vi "Get Broadcast Event.vi"(8 "error in (no error)":errorcluster, 11 "Debug View In":refnum<class "Debug View.lvclass">) -> (0 "error out":errorcluster, 2 "Broadcast Event":refnum<user-event>[](array[refnum]), 3 "Debug View Out":refnum<class "Debug View.lvclass">)   [LabVIEW 2020, in "Debug View.lvclass"]
doc: "Get the broadcast event used to send broadcasts to registered observers."
uses:
  Debug View.lvclass
  Protected/Broadcasting/Broadcast Message Cluster.ctl
  Debug View.lvclass/Debug View.ctl
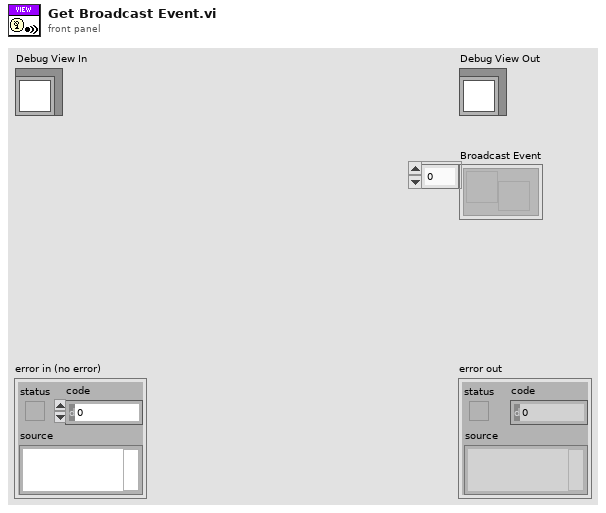
[diagram p1: front panel]
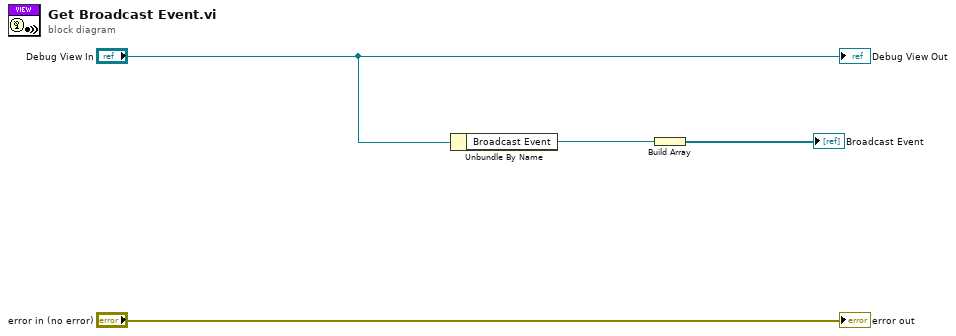
[diagram p0: block diagram]
diagram:
  n1 = Unbundle By Name("Debug View In") -> ("Broadcast Event"=w2:refnum<user-event>)
  n2 = Build Array(w2) -> (→"Broadcast Event":refnum<user-event>[])
  "error out" <- "error in (no error)"
  "Debug View Out" <- "Debug View In"
